vi "OC_SC_Detection.vi"() -> (2 "Open Loop Channels Array":bool[](array[boolean]), 3 "Short Circuit Channels Array":bool[](array[boolean]))   [LabVIEW 2017, in "BOP_VibAPI_6.lvlib"]
uses:
  <vilib>/addons/InsightCM/Devices/Shared/Cms/Fpga/Acquisition/source/subVIs/VibAPI/BOP_VibAPI_6.lvlib
  <vilib>/rvi/eio/common/nirviEmuTemplateMethod_errors.vi
  <vilib>/eio/EIOMethodNode/EIOMethodNode.xnode
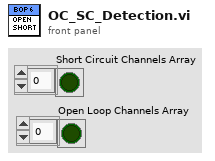
[diagram p1: front panel]
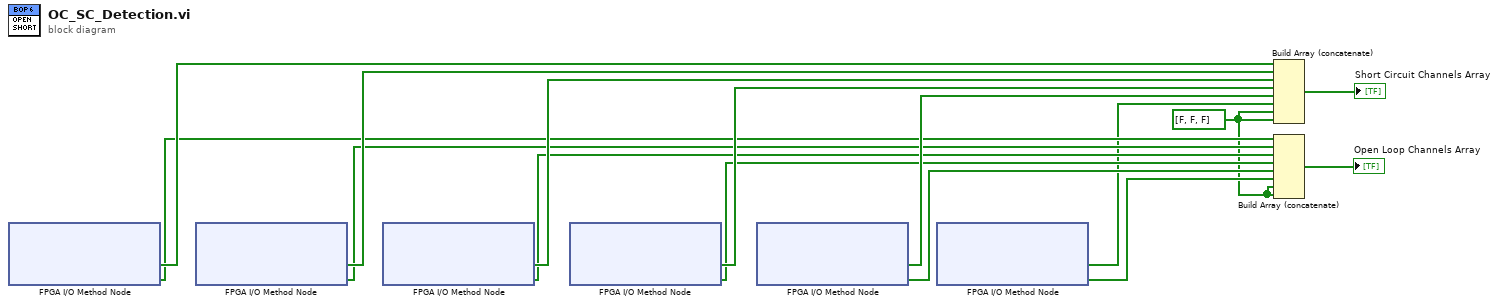
[diagram p0: block diagram]
diagram:
  w3 = bool[] [FALSE, FALSE, FALSE] ("array")
  n1 = xnode "FPGA I/O Method Node"() -> ("Short Circuit"=w15:bool[], "Open Loop"=w10:bool[])  [unwired: 1 in, 1 out]
  n2 = xnode "FPGA I/O Method Node"() -> ("Short Circuit"=w14:bool[], "Open Loop"=w9:bool[])  [unwired: 1 in, 1 out]
  n3 = xnode "FPGA I/O Method Node"() -> ("Short Circuit"=w13:bool[], "Open Loop"=w8:bool[])  [unwired: 1 in, 1 out]
  n4 = xnode "FPGA I/O Method Node"() -> ("Short Circuit"=w12:bool[], "Open Loop"=w7:bool[])  [unwired: 1 in, 1 out]
  n5 = xnode "FPGA I/O Method Node"() -> ("Short Circuit"=w11:bool[], "Open Loop"=w6:bool[])  [unwired: 1 in, 1 out]
  n6 = xnode "FPGA I/O Method Node"() -> ("Short Circuit"=w5:bool[], "Open Loop"=w4:bool[])  [unwired: 1 in, 1 out]
  n7 = Build Array (concatenate)(w15, w14, w13, w12, w11, w5, w3, w3) -> (→"Short Circuit Channels Array":bool[])
  n8 = Build Array (concatenate)(w10, w9, w8, w7, w6, w4, w3, w3) -> (→"Open Loop Channels Array":bool[])
